vi "获取版本名字.vi"() -> (2 "before substring":string)   [LabVIEW 2016]
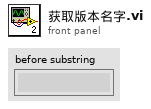
[diagram p1: front panel]
types:
  T1 = enum32{"invalid app kind", "Development System", "Run Time System", "Student Edition", "Embedded LabVIEW", "Evaluation", "Custom"}
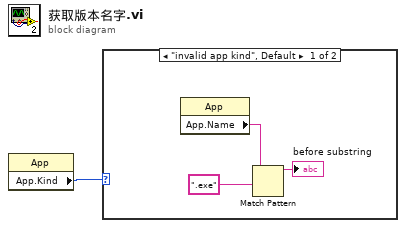
[diagram p0: block diagram]
diagram:
  n1 = property class="App"() -> ("App.Kind"=w1:T1)  [unwired: 2 in, 2 out]
  n2 = case shown="\"invalid app kind\", Default" w1 {
    frame "invalid app kind", Default {
      n3 = property class="App"() -> ("App.Name"=w2:string)  [unwired: 2 in, 2 out]
      n4 = Match Pattern(string=w2, regular expression=".exe") -> (before substring=→"before substring":string)  [unwired: 1 in, 3 out]
    }
    frame "Development System" {
    }
  }
